vi "DHE_ShareNewObs.vi"(4 "exptime (ms)":i32, 6 "async?":bool=TRUE, 8 "error in (no error)":errorcluster) -> (0 "error out":errorcluster, 2 "obsID":string)   [LabVIEW 2016]
uses:
  DBSHAND/private/vis/DatabaseHand_Element_Get(string).vi
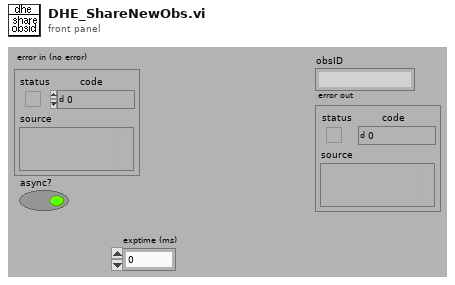
[diagram p1: front panel]
types:
  T1 = typedef "DatabaseHand_RefNum.ctl" = refnum<vi>
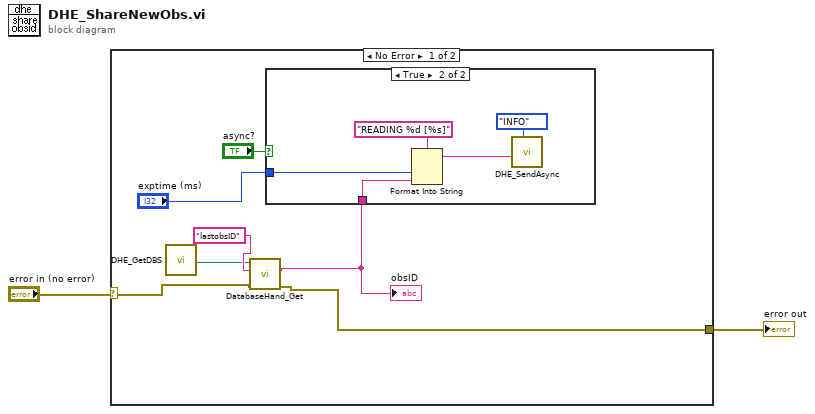
[diagram p0: block diagram]
diagram:
  n1 = case shown="No Error" "error in (no error)" {
    selector: "error in (no error)" -> [w7 w15]
    tunnel: [w6 w15] -> w2
    frame No Error {
      n2 = call "DHE_GetDBS.vi"() -> ("DHE_DBSRef"=w3:T1)  [unwired: 9 out]
      n3 = call-poly "DatabaseHand_Get.vi"("error in (no error)"=w7, "name"="lastobsID", "Database RefNum in"=w3) -> ("error out"=w6:errorcluster, "value"=w4:string)  [unwired: 2 in, 5 out]
      "obsID" <- w4
      n4 = case shown="True" "async?" {
        tunnel: w4 -> [_ w10]
        tunnel: "exptime (ms)" -> [_ w12]
        frame False {
        }
        frame True {
          n5 = Format Into String(format string="READING %d [%s]", w12, w10) -> (resulting string=w11:string)  [unwired: 2 in, 1 out]
          n6 = call "DHE_SendAsync.vi"("type"=enum16{"ERROR", "WARNING", "INFO", "CHANGED"}."INFO", "Message"=w11) -> ()  [unwired: 2 in, 8 out]
        }
      }
    }
    frame Error {
    }
  }
  "error out" <- w2
